vi "HEWH Reset Timer.vi"(0 "Reset Timer (A-D)":bool[](array[boolean]), 1 "Reset Timer (A)":bool, 2 "Reset Timer (B)":bool, 3 "Reset Timer (C)":bool, 4 "Reset Timer (D)":bool, 5 "Error In":errorcluster) -> (14 "Reset D":bool, 15 "Reset C":bool, 16 "Reset B":bool, 17 "Reset A":bool, 19 "Error Out":errorcluster)   [LabVIEW 2014]
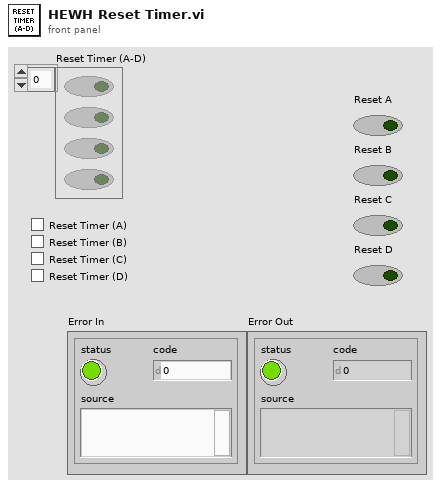
[diagram p1: front panel]
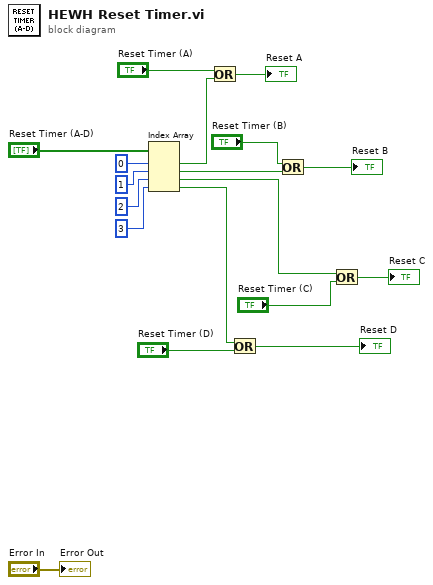
[diagram p0: block diagram]
diagram:
  n1 = Index Array(array="Reset Timer (A-D)", index #1=0 ("index"), index #2=1 ("index"), index #3=2 ("index"), index #4=3 ("index")) -> (element #1=w13:bool, element #2=w11:bool, element #3=w8:bool, element #4=w6:bool)
  n2 = Or(x="Reset Timer (A)", y=w13) -> (x .or. y?=→"Reset A":bool)
  n3 = Or(x=w6, y="Reset Timer (D)") -> (x .or. y?=→"Reset D":bool)
  n4 = Or(x="Reset Timer (B)", y=w11) -> (x .or. y?=→"Reset B":bool)
  n5 = Or(x=w8, y="Reset Timer (C)") -> (x .or. y?=→"Reset C":bool)
  "Error Out" <- "Error In"
